vi "Simple Example.vi"() -> ()   [LabVIEW 2020]
uses:
  C:/GEECS/Developers Version/source/Device Drivers/ThorlabsKCube_InertialMotor/Kinesis/Thorlabs.MotionControl.Controls.dll
  Kinesis/Thorlabs.MotionControl.Controls.dll
  C:/GEECS/Developers Version/source/Device Drivers/ThorlabsKCube_InertialMotor/Kinesis/Thorlabs.MotionControl.KCube.InertialMotorCLI.dll
  Kinesis/Thorlabs.MotionControl.KCube.InertialMotorCLI.dll
panel:
  out "CreateDevice":bool
  in  "KCubeInertialMotorControl":refnum<k24>(container)
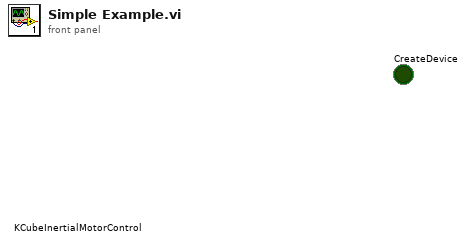
[diagram p1: front panel]
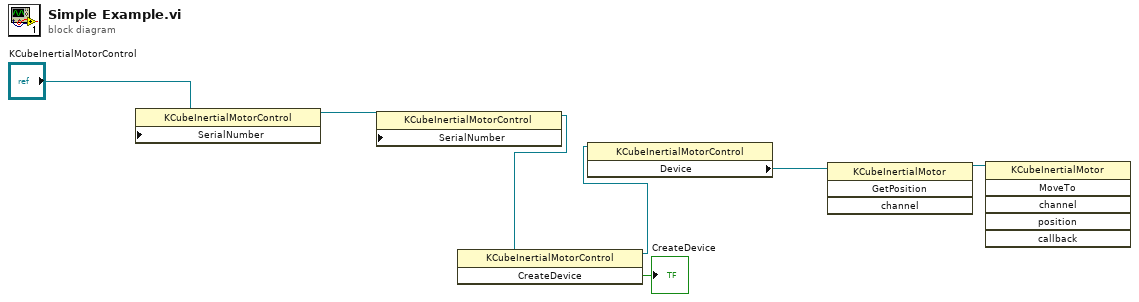
[diagram p0: block diagram]
diagram:
  n1 = property class="KCubeInertialMotorControl" props=["SerialNumber"](reference="KCubeInertialMotorControl") -> (reference out=w6:refnum<k24>)  [unwired: 2 in, 1 out]
  n2 = property class="KCubeInertialMotorControl" props=["SerialNumber"](reference=w6) -> (reference out=w5:refnum<k24>)  [unwired: 2 in, 1 out]
  n3 = invoke class="KCubeInertialMotorControl" method="CreateDevice"(reference=w5) -> (reference out=w3:refnum<k24>, "CreateDevice"=→"CreateDevice":bool)  [unwired: 2 in, 1 out]
  n4 = property class="KCubeInertialMotorControl"(reference=w3) -> ("Device"=w2:refnum<k24>)  [unwired: 1 in, 2 out]
  n5 = invoke class="KCubeInertialMotor" method="GetPosition"(reference=w2) -> (reference out=w1:refnum<k24>)  [unwired: 3 in, 3 out]
  n6 = invoke class="KCubeInertialMotor" method="MoveTo"(reference=w1) -> ()  [unwired: 5 in, 6 out]
